vi "Camera.SaveImg.vi"(8 "error in (no error)":errorcluster, 10 "Path":path, 11 "Camera":refnum<class "Camera.lvclass">) -> (0 "error out":errorcluster, 3 "Camera out":refnum<class "Camera.lvclass">)   [LabVIEW 2013, in "Camera.lvclass"]
doc: "---------------------------------------------------------------\nJKI State Machine Objects™\nhttp://jki.net/state-machine-objects/\nCopyright (C) 2005-2015, JKI <info@jki.net>\nALL RIGHTS RESERVEDJKI State Machine Objects (SMO) 1.0.0.5\nJKI - JKI\nCopyright (c) 2016, JKI"
uses:
  Camera.lvclass
  Program Files (x86)/National Instruments/LabVIEW 2019/user.lib/_OpenG.lib/file/file.llb/Strip Path Extension - Path__ogtk.vi
panel:
  # "For instructions on how to use the JKI State Machine Objects, examples and video tutorials, visit:\nhttp://jki.net/state-machine-objects/\n\nJKI State Machine Objects™\nhttp://jki.net/state-machine-objects/\nCopyright (C) 2005-2015, JKI <info@jki.net>\nALL RIGHTS RESERVED"
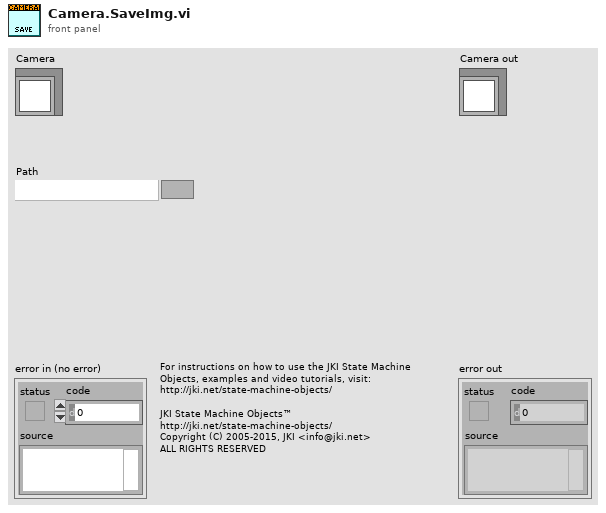
[diagram p1: front panel]
types:
  T1 = typedef "imagedata.ctl" = cluster{"image type":i32, "image depth":i32, "image":u8[], "mask":u8[], "colors":u32[], "Rectangle":cluster{"left":i16, "top":i16, "right":i16, "bottom":i16}}
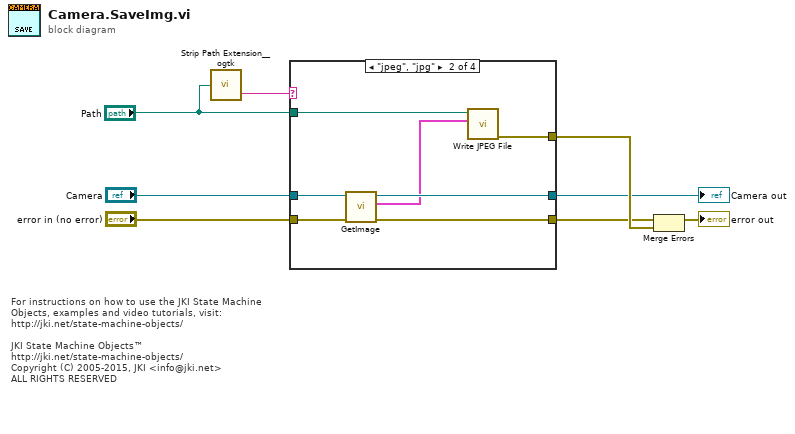
[diagram p0: block diagram]
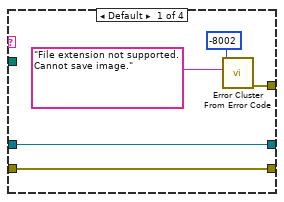
[diagram p2: hidden frame]
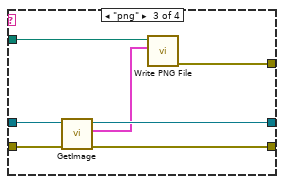
[diagram p3: hidden frame]
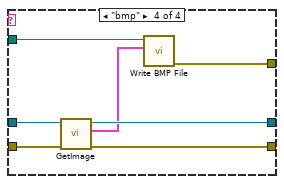
[diagram p4: hidden frame]
diagram:
  # "For instructions on how to use the JKI State Machine Objects, examples and video tutorials, visit:\nhttp://jki.net/state-machine-objects/\n\nJKI State Machine Objects™\nhttp://jki.net/state-machine-objects/\nCopyright (C) 2005-2015, JKI <info@jki.net>\nALL RIGHTS RESERVED"
  n1 = call-poly "Strip Path Extension__ogtk.vi"("path"="Path") -> ("extension"=w8:string)  [unwired: 1 out]
  n2 = case shown="\"jpeg\", \"jpg\"" w8 {
    tunnel: "Path" -> [_ w20 w27 w34]
    tunnel: [w13 w19 w26 w33] -> w7
    tunnel: "Camera" -> [w11 w18 w25 w32]
    tunnel: "error in (no error)" -> [w10 w17 w24 w31]
    tunnel: [w11 w15 w22 w30] -> w3
    tunnel: [w10 w16 w23 w29] -> w2
    frame Default {
      n3 = call <vilib>:"Error Cluster From Error Code.vi"("error message (\"\")"="File extension not supported. Cannot save image.", "error code (0)"=-8002) -> ("error out"=w13:errorcluster)  [unwired: 7 in]
    }
    frame "jpeg", "jpg" {
      n4 = call "GetImage.vi"("error in (no error)"=w17, "Camera"=w18) -> ("error out"=w16:errorcluster, "image data"=w14:T1, "Camera out"=w15:refnum<class "Camera.lvclass">)  [unwired: 7 in]
      n5 = call <vilib>:"Write JPEG File.vi"("image data"=w14, "path to JPEG file"=w20) -> ("error out"=w19:errorcluster)  [unwired: 8 in, 1 out]
    }
    frame "png" {
      n6 = call "GetImage.vi"("error in (no error)"=w24, "Camera"=w25) -> ("error out"=w23:errorcluster, "image data"=w21:T1, "Camera out"=w22:refnum<class "Camera.lvclass">)  [unwired: 7 in]
      n7 = call <vilib>:"Write PNG File.vi"("image data"=w21, "path to PNG file"=w27) -> ("error out"=w26:errorcluster)  [unwired: 8 in, 1 out]
    }
    frame "bmp" {
      n8 = call "GetImage.vi"("error in (no error)"=w31, "Camera"=w32) -> ("error out"=w29:errorcluster, "image data"=w28:T1, "Camera out"=w30:refnum<class "Camera.lvclass">)  [unwired: 7 in]
      n9 = call <vilib>:"Write BMP File.vi"("image data"=w28, "path to BMP file"=w34) -> ("error out"=w33:errorcluster)  [unwired: 8 in, 1 out]
    }
  }
  "Camera out" <- w3
  n10 = Merge Errors(w2, w7) -> (→"error out":errorcluster)
